vi "Message decoding.vi"(8 "error in (no error)":errorcluster, 10 "Message":string, 11 "Kasli Listener in":refnum<class "Kasli Listener.lvclass">) -> (0 "error out":errorcluster, 2 "Message decoded":T1, 3 "Kasli Listener out":refnum<class "Kasli Listener.lvclass">)   [LabVIEW 2020, in "Kasli Listener and Writer.lvlib" / "Kasli Listener.lvclass"]
uses:
  Kasli Listener.lvclass
  System uServices/TCP Writer/TCP Writer/TCP Message Internal Composition.ctl
  System uServices/TCP Writer/TCP Writer/TCP Writer.lvclass
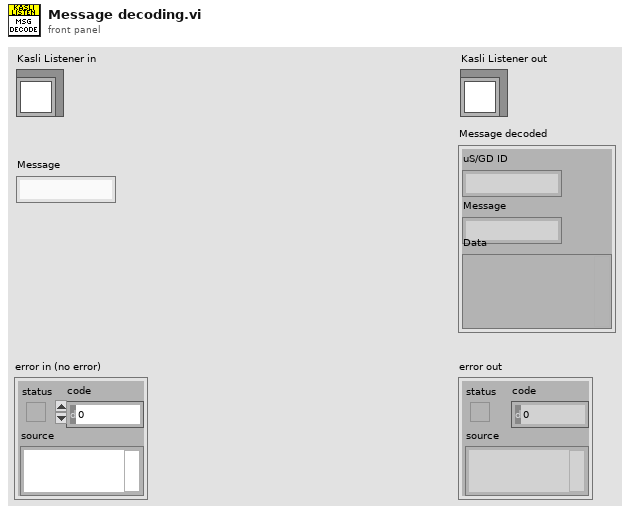
[diagram p1: front panel]
types:
  T1 = typedef "TALOS.lvlib/TCP Writer.lvlib/TCP Writer.lvclass/TCP Message Internal Composition.ctl" = cluster{"uS/GD ID":string, "Message":string, "Data":variant}
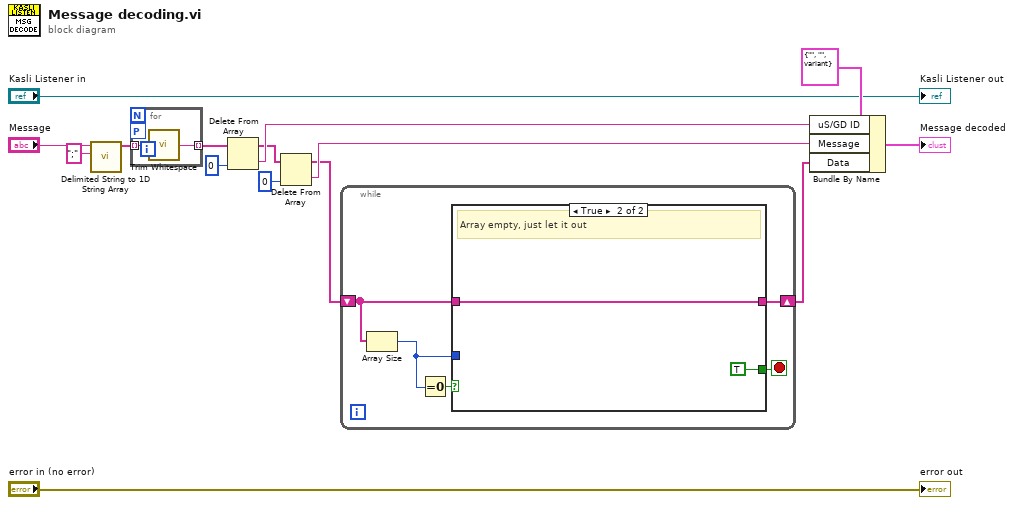
[diagram p0: block diagram]
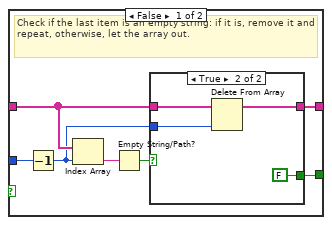
[diagram p2: hidden frame]
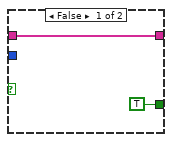
[diagram p3: hidden frame]
diagram:
  n1 = call <vilib>:"Delimited String to 1D String Array.vi"("delimiter"=";", "delimited string"="Message") -> ("string array"=w9:string[])  [unwired: 9 in]
  n2 = for {
    tunnel: w9 -> [w17] mode=indexing
    tunnel: [w16] -> w8 mode=indexing
    workers-P: _ -> [_]
    n3 = call <vilib>:"Trim Whitespace.vi"("string"=w17) -> ("trimmed string"=w16:string)  [unwired: 1 in]
  }
  n4 = Delete From Array(array=w8, index=0) -> (deleted portion=w6:string, array with subset deleted=w5:string[])  [unwired: 1 in]
  n5 = Delete From Array(array=w5, index=0) -> (deleted portion=w3:string, array with subset deleted=w2:string[])  [unwired: 1 in]
  n6 = while {
    shift-right: [w19] -> w1
    shift-left: w2 -> [w20]
    stop <- w18 stop-if-true
    n7 = Array Size(array=w20) -> (size(s)=w22:i32)
    n8 = Equal To 0?(x=w22) -> (x = 0?=w21:bool)
    n9 = case shown="True" w21 {
      tunnel: w22 -> [w29 _]
      tunnel: w20 -> [w25 w37]
      tunnel: [w26 w37] -> w19
      tunnel: [w24 TRUE] -> w18
      frame False {
        # "Check if the last item is an empty string: if it is, remove it and repeat, otherwise, let the array out."
        n10 = Decrement(x=w29) -> (x-1=w23:i32)
        n11 = Index Array(array=w25, index=w23) -> (element=w28:string)
        n12 = Empty String/Path?(string/path=w28) -> (empty?=w27:bool)
        n13 = case shown="True" w27 {
          tunnel: [w31 w33] -> w26
          tunnel: w25 -> [w31 w35]
          tunnel: [TRUE FALSE] -> w24
          tunnel: w23 -> [_ w34]
          frame False {
          }
          frame True {
            n14 = Delete From Array(array=w35, index=w34) -> (array with subset deleted=w33:string[])  [unwired: 1 in, 1 out]
          }
        }
      }
      frame True {
        # "Array empty, just let it out"
      }
    }
  }
  n15 = Bundle By Name(cluster=T1 {"uS/GD ID"="", "Message"="", "Data"=variant} ("Message decoded"), "uS/GD ID"=w6, "Message"=w3, "Data"=w1) -> (→"Message decoded":T1)
  "error out" <- "error in (no error)"
  "Kasli Listener out" <- "Kasli Listener in"
